vi "Assert Cal Attendance Result.vi"   [LabVIEW 2015, in "Admin_Actor.lvlib" / "AttendRecord.lvclass"]
uses:
  AttendRecord.lvclass
  Setting/g_setting.vi
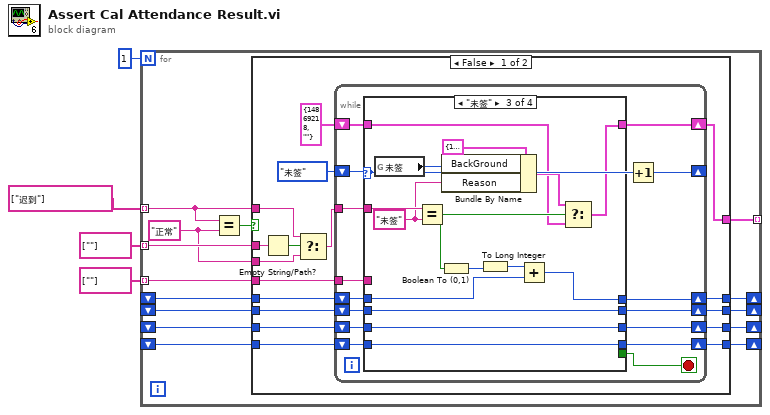
[diagram p0: block diagram]
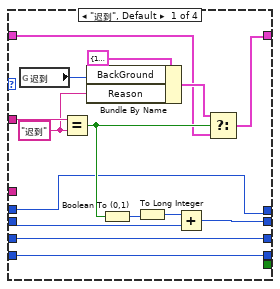
[diagram p2: hidden frame]
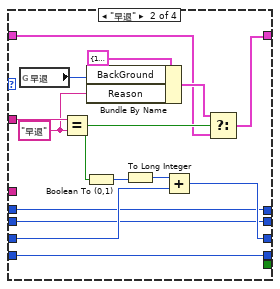
[diagram p3: hidden frame]
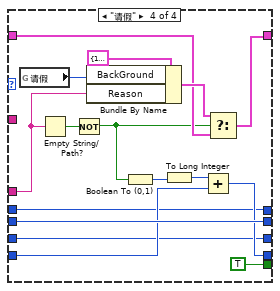
[diagram p4: hidden frame]
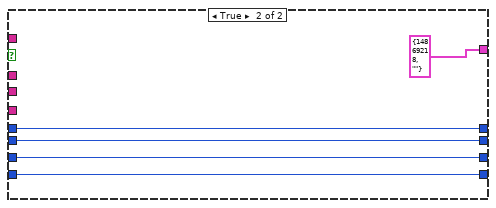
[diagram p5: hidden frame]
diagram:
  n1 = for {
    N: 1 -> [_]
    tunnel: string[] ["迟到"] ("Calendances(\"\")") -> [w14] mode=indexing
    tunnel: string[] [""] ("TimeTables(\"\")") -> [w16] mode=indexing
    tunnel: string[] [""] ("ExcuseNotes(\"\")") -> [w15] mode=indexing
    tunnel: [w17] -> _ mode=indexing
    shift-right: [w9] -> _
    shift-left: _ -> [w12]
    shift-right: [w8] -> _
    shift-left: _ -> [w11]
    shift-right: [w7] -> _
    shift-left: _ -> [w10]
    shift-right: [w5] -> _
    shift-left: _ -> [w6]
    w13 = "正常" ("y")
    n2 = Equal?(x=w14, y=w13) -> (x = y?=w18:bool)
    n3 = case shown="False" w18 {
      tunnel: [w29 cluster{"BackGround":u32, "Reason":string} {"BackGround"=14869218, "Reason"=""} ("Display")] -> w17
      tunnel: w16 -> [w28 _]
      tunnel: w15 -> [w30 _]
      tunnel: w14 -> [w26 _]
      tunnel: w13 -> [w21 _]
      tunnel: w12 -> [w34 w115]
      tunnel: w11 -> [w33 w114]
      tunnel: w10 -> [w32 w113]
      tunnel: [w24 w115] -> w9
      tunnel: [w23 w114] -> w8
      tunnel: [w22 w113] -> w7
      tunnel: w6 -> [w20 w112]
      tunnel: [w19 w112] -> w5
      frame False {
        n4 = Empty String/Path?(string/path=w28) -> (empty?=w27:bool)
        n5 = Select(t=w26, s=w27, f=w21) -> (s? t:f=w25:string)
        n6 = while {
          tunnel: w25 -> [w50]
          shift-right: [w49] -> w29
          shift-left: cluster{"BackGround":u32, "Reason":string} {"BackGround"=14869218, "Reason"=""} ("Display") -> [w48]
          shift-right: [w46] -> _
          shift-left: enum16{"迟到", "早退", "未签", "请假"}."未签" -> [w47]
          shift-right: [w42] -> w24
          shift-left: w34 -> [w45]
          shift-right: [w41] -> w23
          shift-left: w33 -> [w44]
          shift-right: [w40] -> w22
          shift-left: w32 -> [w43]
          tunnel: w30 -> [w39]
          shift-right: [w36] -> w19
          shift-left: w20 -> [w37]
          stop <- w38 stop-if-true
          n7 = case shown="\"未签\"" w47 {
            tunnel: w50 -> [w65 w80 w95 _]
            tunnel: [w60 w75 w90 w108] -> w49
            tunnel: w48 -> [w54 w71 w86 w105]
            tunnel: w45 -> [w58 w68 w85 w104]
            tunnel: w44 -> [w53 w70 w81 w98]
            tunnel: w43 -> [w52 w67 w84 w100]
            tunnel: [w55 w68 w85 w104] -> w42
            tunnel: [w53 w69 w81 w98] -> w41
            tunnel: [w52 w67 w84 w99] -> w40
            tunnel: w39 -> [_ _ _ w103]
            tunnel: [_ _ _ TRUE] -> w38
            tunnel: w37 -> [w51 w66 w83 w96]
            tunnel: [w51 w66 w82 w96] -> w36
            frame "迟到", Default {
              w62 = "迟到" ("y")
              n8 = global read "g_setting.vi" "迟到"() -> (w63:u32)
              n9 = Equal?(x=w65, y=w62) -> (x = y?=w59:bool)
              n10 = Bundle By Name(cluster=cluster{"BackGround":u32, "Reason":string} {"BackGround"=14869218, "Reason"=""} ("Display"), "BackGround"=w63, "Reason"=w62) -> (w61:cluster{"BackGround":u32, "Reason":string})
              n11 = Boolean To (0,1)(Boolean=w59) -> (0, 1=w57:i16)
              n12 = To Long Integer(number=w57) -> (32bit integer=w56:i32)
              n13 = Add(x=w56, y=w58) -> (x+y=w55:i32)
              n14 = Select(t=w61, s=w59, f=w54) -> (s? t:f=w60:cluster{"BackGround":u32, "Reason":string})
            }
            frame "早退" {
              w77 = "早退" ("y")
              n15 = global read "g_setting.vi" "早退"() -> (w78:u32)
              n16 = Equal?(x=w80, y=w77) -> (x = y?=w74:bool)
              n17 = Boolean To (0,1)(Boolean=w74) -> (0, 1=w73:i16)
              n18 = Bundle By Name(cluster=cluster{"BackGround":u32, "Reason":string} {"BackGround"=14869218, "Reason"=""} ("Display"), "BackGround"=w78, "Reason"=w77) -> (w76:cluster{"BackGround":u32, "Reason":string})
              n19 = To Long Integer(number=w73) -> (32bit integer=w72:i32)
              n20 = Add(x=w72, y=w70) -> (x+y=w69:i32)
              n21 = Select(t=w76, s=w74, f=w71) -> (s? t:f=w75:cluster{"BackGround":u32, "Reason":string})
            }
            frame "未签" {
              w92 = "未签" ("y")
              n22 = global read "g_setting.vi" "未签"() -> (w93:u32)
              n23 = Equal?(x=w95, y=w92) -> (x = y?=w89:bool)
              n24 = Boolean To (0,1)(Boolean=w89) -> (0, 1=w88:i16)
              n25 = Bundle By Name(cluster=cluster{"BackGround":u32, "Reason":string} {"BackGround"=14869218, "Reason"=""} ("Display"), "BackGround"=w93, "Reason"=w92) -> (w91:cluster{"BackGround":u32, "Reason":string})
              n26 = To Long Integer(number=w88) -> (32bit integer=w87:i32)
              n27 = Add(x=w87, y=w83) -> (x+y=w82:i32)
              n28 = Select(t=w91, s=w89, f=w86) -> (s? t:f=w90:cluster{"BackGround":u32, "Reason":string})
            }
            frame "请假" {
              n29 = global read "g_setting.vi" "请假"() -> (w110:u32)
              n30 = Empty String/Path?(string/path=w103) -> (empty?=w102:bool)
              n31 = Not(x=w102) -> (.not. x?=w101:bool)
              n32 = Bundle By Name(cluster=cluster{"BackGround":u32, "Reason":string} {"BackGround"=14869218, "Reason"=""} ("Display"), "BackGround"=w110, "Reason"=w103) -> (w109:cluster{"BackGround":u32, "Reason":string})
              n33 = Boolean To (0,1)(Boolean=w101) -> (0, 1=w107:i16)
              n34 = To Long Integer(number=w107) -> (32bit integer=w106:i32)
              n35 = Add(x=w106, y=w100) -> (x+y=w99:i32)
              n36 = Select(t=w109, s=w101, f=w105) -> (s? t:f=w108:cluster{"BackGround":u32, "Reason":string})
            }
          }
          n37 = Increment(x=w47) -> (x+1=w46:enum16{"迟到", "早退", "未签", "请假"})
        }
      }
      frame True {
      }
    }
  }
